vi "Swerve Wheels.vi"(0 "Yaw":dbl, 1 "Robot Width":dbl, 2 "Y Command":dbl, 3 "X Command":dbl, 4 "Z Command":dbl, 5 "Rot. Point X":dbl, 6 "Robot  Length":dbl, 7 "Rot. Point Y":dbl) -> (24 "output cluster":T1)   [LabVIEW 2019]
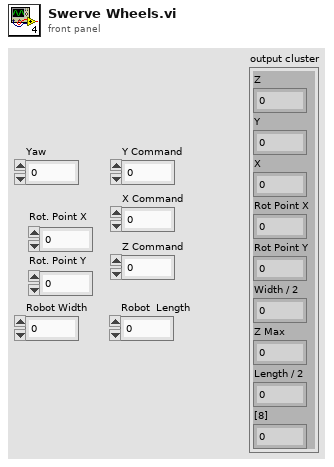
[diagram p1: front panel]
types:
  T1 = cluster{"Z":dbl, "Y":dbl, "X":dbl, "Rot Point X":dbl, "Rot Point Y":dbl, "Width / 2":dbl, "Z Max":dbl, "Length / 2":dbl, "[8]":dbl}
  T2 = cluster{"[0]":dbl, "[1]":dbl, "[2]":dbl, "[3]":dbl, "[4]":dbl, "[5]":dbl, "[6]":dbl, "[7]":dbl, "[8]":dbl}
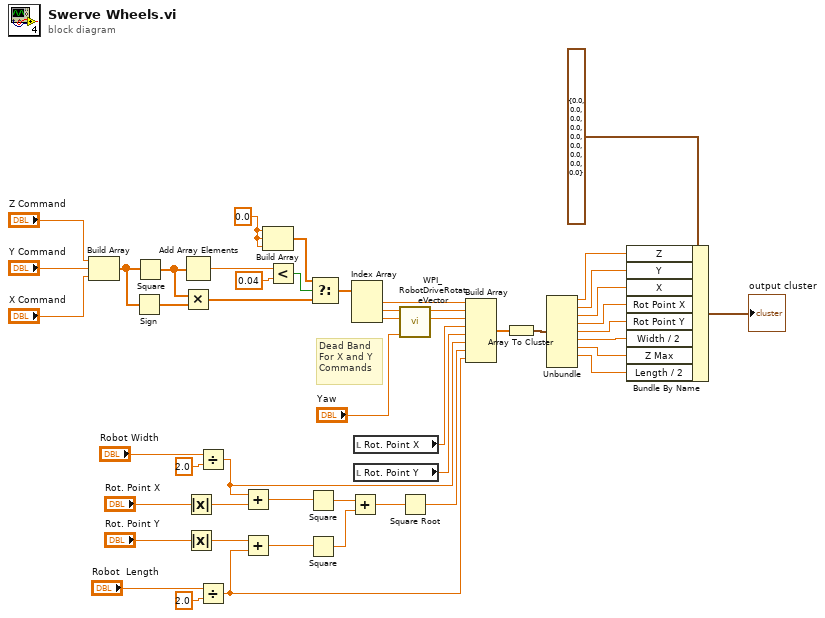
[diagram p0: block diagram]
diagram:
  w26 = 0.0 ("element")
  # "Dead Band \nFor X and Y\nCommands"
  n1 = Build Array("Z Command", "Y Command", "X Command") -> (w22:dbl[])
  n2 = Sign(1:w22) -> (0:w25:dbl[])
  n3 = Square(x=w22) -> (x^2=w24:dbl[])
  n4 = Add Array Elements(numeric array=w24) -> (sum=w30:dbl)
  n5 = Multiply(x=w24, y=w25) -> (x*y=w23:dbl[])
  n6 = Absolute Value(x="Rot. Point X") -> (abs(x)=w49:dbl)
  n7 = Absolute Value(x="Rot. Point Y") -> (abs(x)=w47:dbl)
  n8 = Divide(x="Robot Width", y=2.0) -> (x/y=w37:dbl)
  n9 = Divide(x="Robot  Length", y=2.0) -> (x/y=w21:dbl)
  n10 = Add(x=w37, y=w49) -> (x+y=w48:dbl)
  n11 = Add(x=w47, y=w21) -> (x+y=w46:dbl)
  n12 = Build Array(w26, w26, w26) -> (w27:dbl[])
  n13 = Less?(x=w30, y=0.04 ("x")) -> (x < y?=w28:bool)
  n14 = Square(x=w48) -> (x^2=w44:dbl)
  n15 = Square(x=w46) -> (x^2=w45:dbl)
  n16 = Select(t=w27, s=w28, f=w23) -> (s? t:f=w34:dbl[])
  n17 = Add(x=w44, y=w45) -> (x+y=w43:dbl)
  n18 = Index Array(array=w34) -> (element #1=w32:dbl, element #2=w35:dbl, element #3=w38:dbl)  [unwired: 3 in]
  n19 = local read "Rot. Point X"() -> (w14:dbl)
  n20 = local read "Rot. Point Y"() -> (w13:dbl)
  n21 = call <vilib>:"WPI_RobotDriveRotateVector.vi"("Angle"="Yaw", "X"=w38, "Y"=w35) -> ("X'"=w33:dbl, "Y'"=w31:dbl)  [unwired: 7 out]
  n22 = Square Root(x=w43) -> (sqrt(x)=w36:dbl)
  n23 = Build Array(w32, w31, w33, w14, w13, w37, w36, w21) -> (w3:dbl[])
  n24 = Array To Cluster(array=w3) -> (cluster=w4:T2)
  n25 = Unbundle(w4) -> ("[0]"=w12:dbl, "[1]"=w11:dbl, "[2]"=w10:dbl, "[3]"=w9:dbl, "[4]"=w8:dbl, "[5]"=w7:dbl, "[6]"=w6:dbl, "[7]"=w5:dbl)  [unwired: 1 out]
  n26 = Bundle By Name(cluster=T1 {"Z"=0.0, "Y"=0.0, "X"=0.0, "Rot Point X"=0.0, "Rot Point Y"=0.0, "Width / 2"=0.0, "Z Max"=0.0, "Length / 2"=0.0, "[8]"=0.0} ("output cluster 2"), "Z"=w12, "Y"=w11, "X"=w10, "Rot Point X"=w9, "Rot Point Y"=w8, "Width / 2"=w7, "Z Max"=w6, "Length / 2"=w5) -> (→"output cluster":T1)
